vi "Initialize.vi"(8 "error in (no error)":errorcluster, 9 "Marca":string, 10 "Puerto Com":refnum<visa-resource-name>, 11 "object in":refnum<class "Simulado.lvclass">) -> (0 "error out":errorcluster, 3 "object out":refnum<class "Simulado.lvclass">)   [LabVIEW 2020, in "Simulado.lvclass"]
uses:
  Simulado.lvclass
  Simulado.lvclass/Simulado.ctl
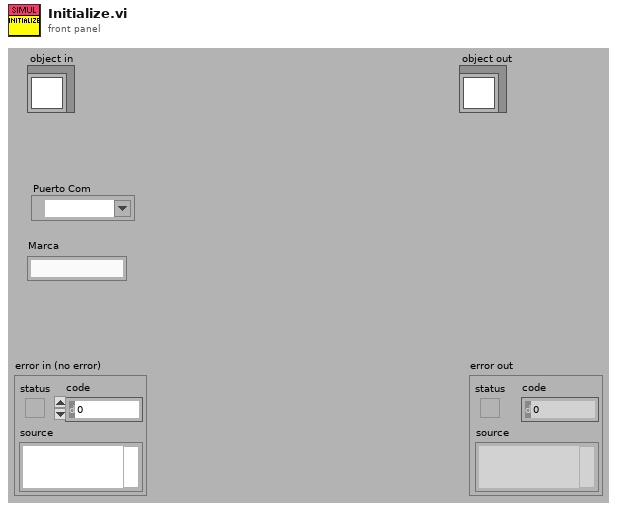
[diagram p1: front panel]
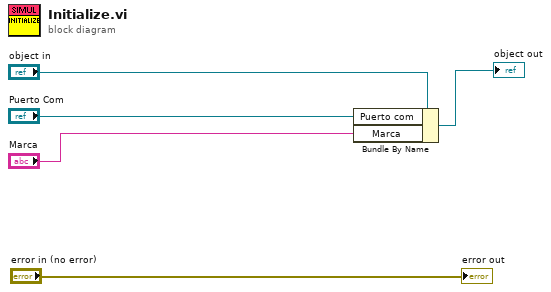
[diagram p0: block diagram]
diagram:
  n1 = Bundle By Name(cluster="object in", "Puerto com"="Puerto Com", "Marca"="Marca") -> (→"object out":refnum<class "Simulado.lvclass">)
  "error out" <- "error in (no error)"
